vi "niDAQmx Write.vi"   [LabVIEW 2021, in "Session Management niDAQmx.lvlib" / "Session Factory.lvclass"]
doc: "Writes samples to the task or virtual channels you specify. The instances of this polymorphic VI specify the format of the samples to write, whether to write one or multiple samples, and whether to write to one or multiple channels."
uses:
  Session Factory.lvclass
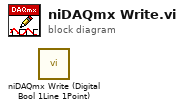
[diagram p0: block diagram]
diagram:
  n1 = call "niDAQmx Write (Digital Bool 1Line 1Point).vi"() -> ()  [unwired: 13 in, 3 out]
